vi "Update Table Step Done by Index.vi"(8 "error in (no error)":errorcluster, 10 "Index":i64, 11 "Kitchen Actor in":refnum<class "Kitchen Actor.lvclass">) -> (0 "error out":errorcluster, 3 "Kitchen Actor out":refnum<class "Kitchen Actor.lvclass">)   [LabVIEW 2021, in "Kitchen Actor.lvlib" / "Kitchen Actor.lvclass"]
uses:
  Kitchen Actor.lvclass
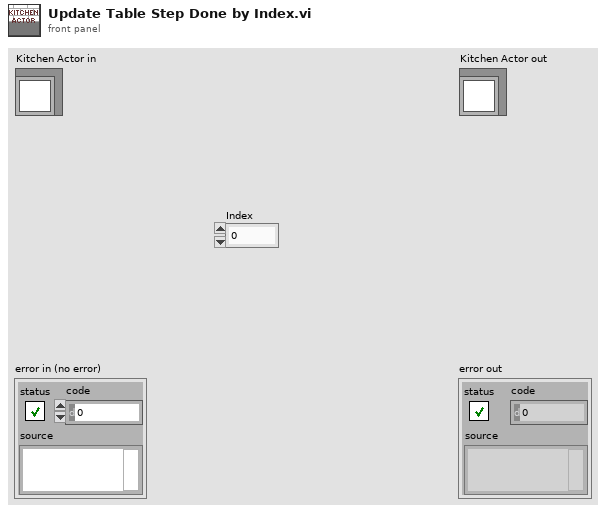
[diagram p1: front panel]
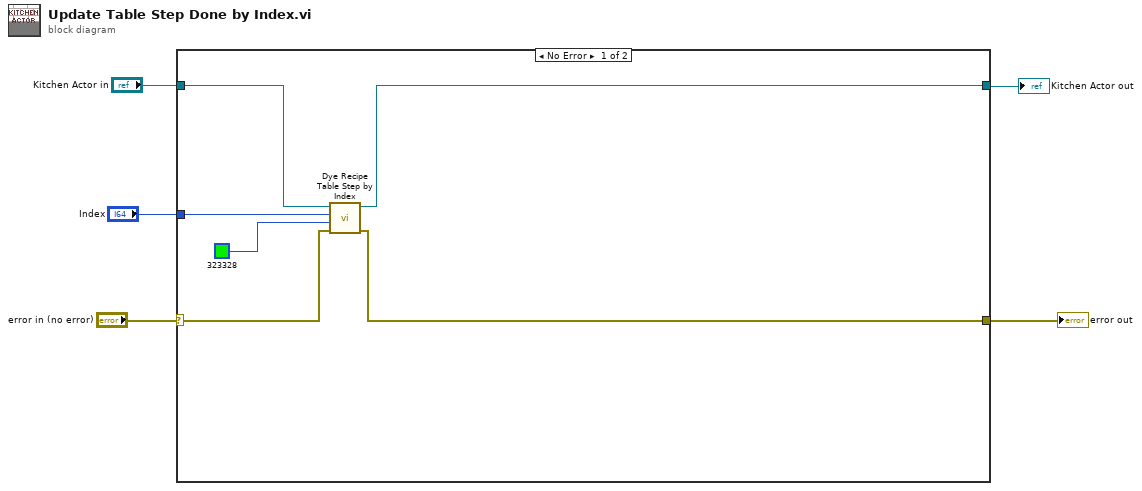
[diagram p0: block diagram]
diagram:
  n1 = case shown="No Error" "error in (no error)" {
    selector: "error in (no error)" -> [w8 w12]
    tunnel: [w7 w12] -> w4
    tunnel: "Kitchen Actor in" -> [w11 w13]
    tunnel: [w6 w13] -> w2
    tunnel: "Index" -> [w10 _]
    frame No Error {
      n2 = call-dynamic "Dye Recipe Table Step by Index.vi"("error in (no error)"=w8, "Dye Color"=u32 323328, "Index"=w10, "Kitchen Actor in"=w11) -> ("error out"=w7:errorcluster, "Kitchen Actor out"=w6:refnum<class "Kitchen Actor.lvclass">)  [unwired: 6 in]
    }
    frame Error {
    }
  }
  "error out" <- w4
  "Kitchen Actor out" <- w2
